vi "Distance.vi"(1 "Array2":u32[](array[numeric]), 2 "Array1":u32[](array[numeric])) -> (0 "Distance":dbl)   [LabVIEW 2020]
panel:
  # "Ευκλέιδια απόσταση δύο διανυσμάτων"
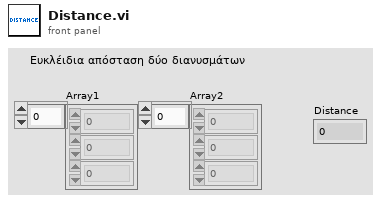
[diagram p1: front panel]
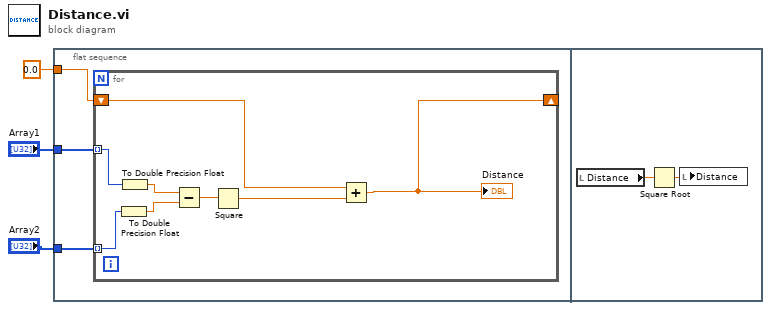
[diagram p0: block diagram]
diagram:
  n1 = flat-sequence {
    tunnel: "Array1" -> [w6]
    tunnel: "Array2" -> [w5]
    tunnel: 0.0 ("Distance") -> [w4]
    frame #0 {
      n2 = for {
        tunnel: w6 -> [w10] mode=indexing
        tunnel: w5 -> [w7] mode=indexing
        shift-right: [w11] -> _
        shift-left: w4 -> [w12]
        n3 = To Double Precision Float(number=w7) -> (double precision float=w8:dbl)
        n4 = To Double Precision Float(number=w10) -> (double precision float=w9:dbl)
        n5 = Subtract(x=w9, y=w8) -> (x-y=w14:dbl)
        n6 = Square(x=w14) -> (x^2=w13:dbl)
        n7 = Add(x=w12, y=w13) -> (x+y=w11:dbl)
        "Distance" <- w11
      }
    }
    frame #1 {
      n8 = local read "Distance"() -> (w16:dbl)
      n9 = Square Root(x=w16) -> (sqrt(x)=w15:dbl)
      n10 = local write "Distance"(w15) -> ()
    }
  }
